vi "Voltage_Current.vi"() -> ()   [LabVIEW 2012]
uses:
  <instrlib>/Tektronix PWS4XXX Series/Tektronix PWS4XXX Series.lvlib
  <instrlib>/Tektronix DMM4020/Tektronix DMM4020.lvlib
panel:
  in  "stop":bool
  in  "Tab Control":T1(tab)
  in  "Step":dbl
  in  "Umin, V":dbl
  in  "Umax, V":dbl
  out "I, A":dbl format="%#.6f"
  out "U, V":dbl
  out "Current-Voltage Curve":cluster{dbl[], dbl[]}(graph)
  in  "Step, s":dbl
  in  "Seconds":dbl
  in  "Minutes":dbl
  in  "Hours":dbl
  in  "Value (V/A)":dbl format="%.2f"
  in  "Fixed function":u16(ring) items=["Voltage", "Current"]
  in  "Measurement Function":u16(ring) items=["DC Volts", "AC Volts", "DC Current", "AC Current", "2-Wire Resistance", "4-Wire Resistance", "Frequency", "AC and DC rms Current", "AC and DC rms Volts", "Continuity", "Diode"]
  out "Present value":dbl format="%#.6f"
  out "Unit":string
  out "Current-Voltage Curve 2":cluster{dbl[], dbl[]}(graph)
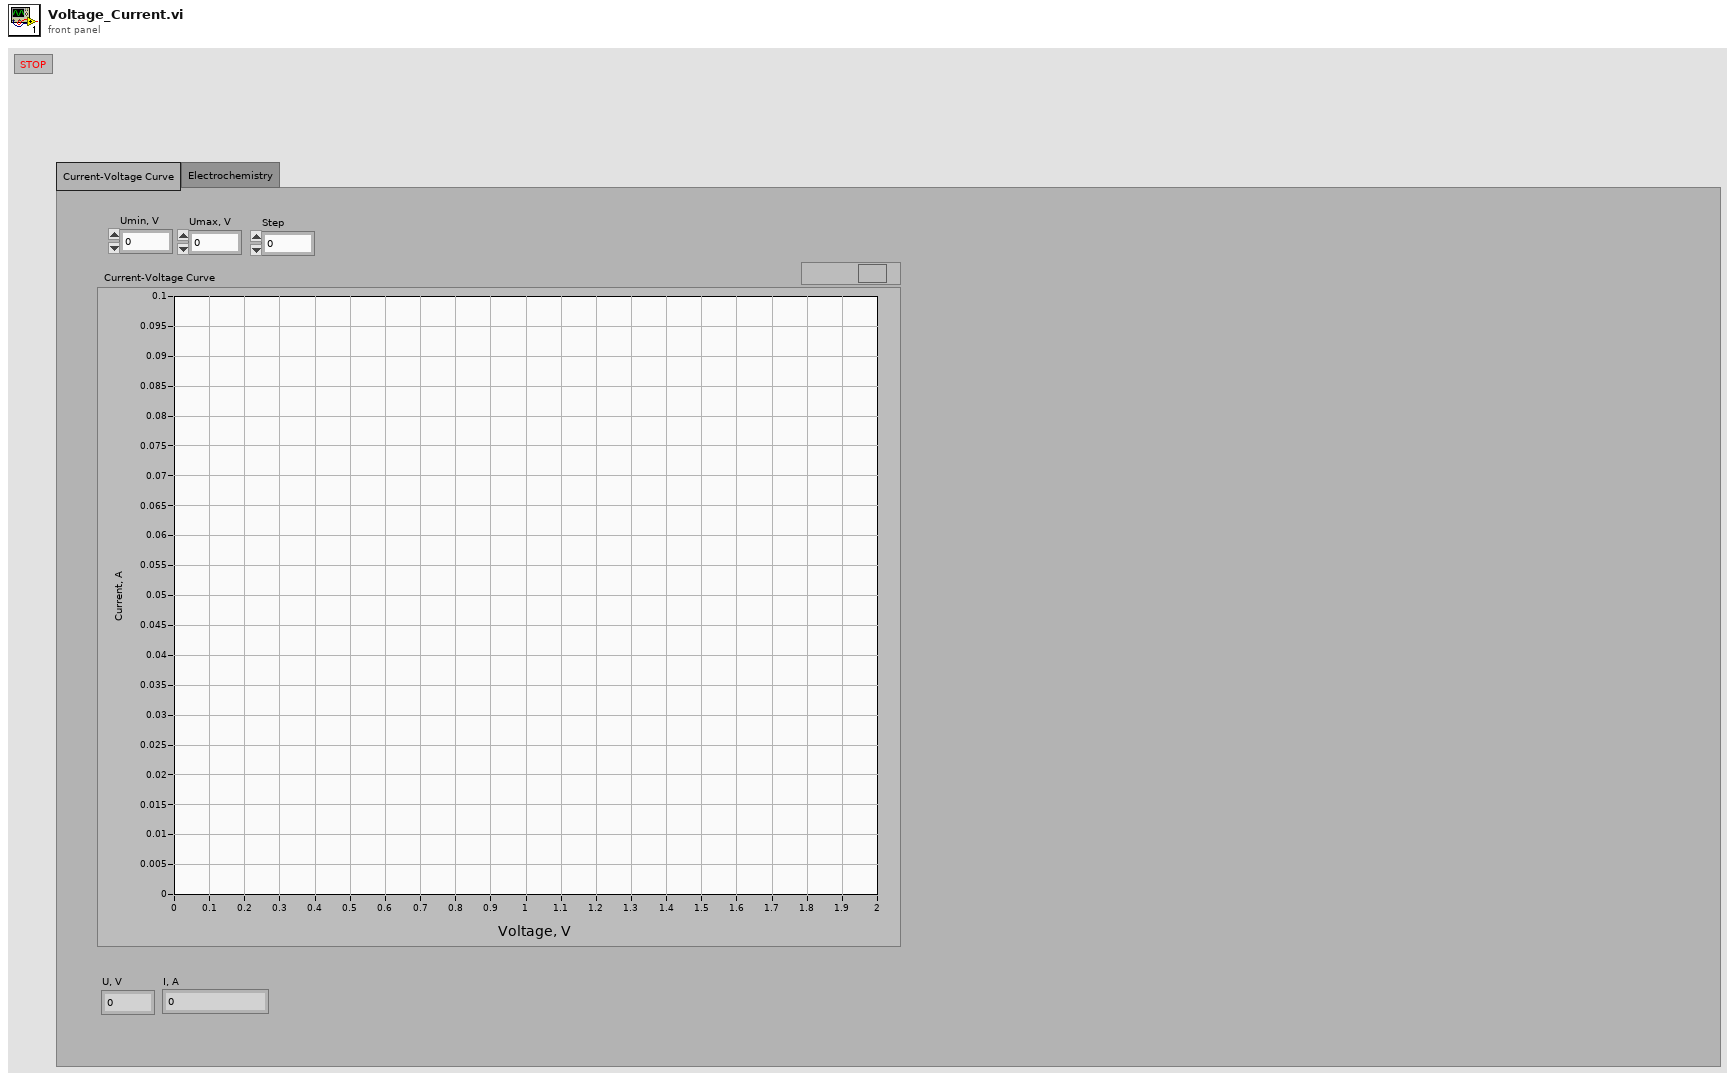
[diagram p1: front panel]
types:
  T1 = enum32{"Current-Voltage Curve", "Electrochemistry"}
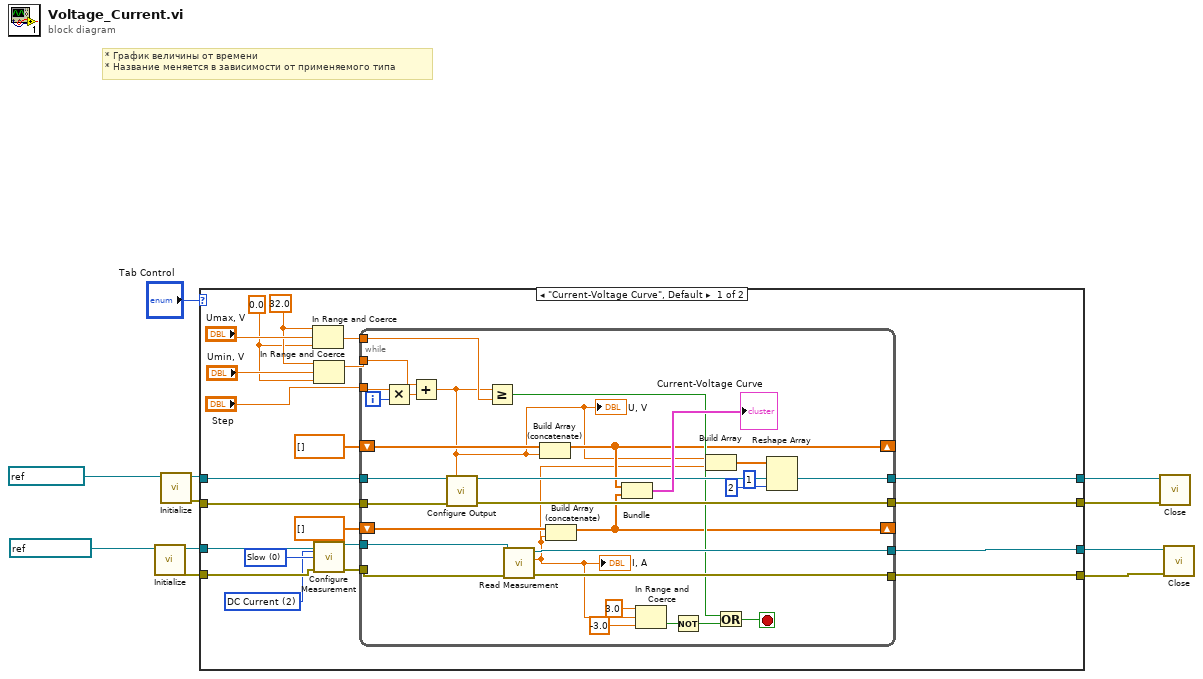
[diagram p0: block diagram]
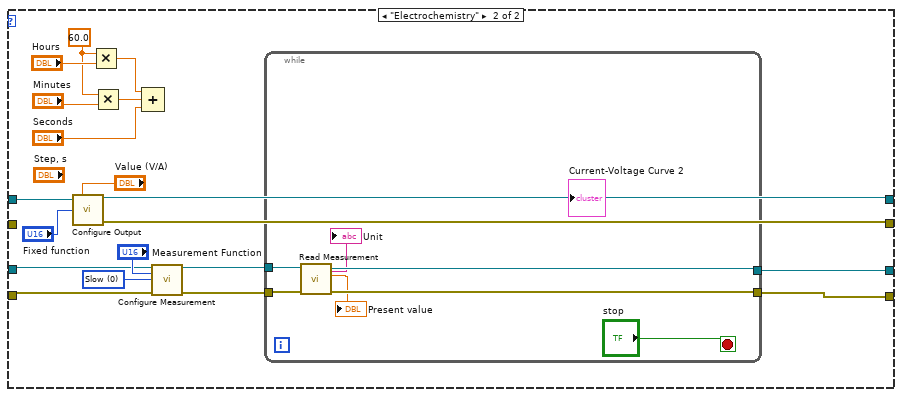
[diagram p2: hidden frame]
diagram:
  # "* График величины от времени\n* Название меняется в зависимости от применяемого типа"
  n1 = call <instrlib>:"Initialize.vi"("VISA resource name"=refnum<visa-resource-name> "DMM4020") -> ("error out"=w8:errorcluster, "VISA resource name out"=w9:refnum<visa-resource-name>)  [unwired: 9 in]
  n2 = call <instrlib>:"Initialize.vi"("VISA resource name"=refnum<visa-resource-name> "PWS4323") -> ("error out"=w2:errorcluster, "VISA resource name out"=w3:refnum<visa-resource-name>)  [unwired: 9 in]
  n3 = case shown="\"Current-Voltage Curve\", Default" "Tab Control" {
    tunnel: w3 -> [w25 w74]
    tunnel: w2 -> [w24 _]
    tunnel: w9 -> [w16 w67]
    tunnel: w8 -> [w15 w66]
    tunnel: [w23 w71] -> w7
    tunnel: [w22 w70] -> w6
    tunnel: [w21 w62] -> w5
    tunnel: [w20 w63] -> w4
    frame "Current-Voltage Curve", Default {
      w17 = u16 0 items=["Slow", "Medium", "Fast"] ("Measurement Rate (0: Slow)")
      w14 = u16 2 items=["DC Volts", "AC Volts", "DC Current", "AC Current", "2-Wire Resistance", "4-Wire Resistance", "Frequency", "AC and DC rms Current", "AC and DC rms Volts", "Continuity", "Diode"] ("Measurement Function (0: DC Volts)")
      w29 = 0.0 ("lower limit")
      w30 = 32.0 ("upper limit")
      n4 = In Range and Coerce(upper limit=w30, x="Umax, V", lower limit=w29) -> (coerced(x)=w26:dbl)  [unwired: 1 out]
      n5 = In Range and Coerce(upper limit=w30, x="Umin, V", lower limit=w29) -> (coerced(x)=w27:dbl)  [unwired: 1 out]
      n6 = call <instrlib>:"Configure Measurement.vi"("VISA resource name"=w16, "Measurement Function (0: DC Volts)"=w14, "Measurement Rate (0: Slow)"=w17, "error in (no error)"=w15) -> ("VISA resource name out"=w13:refnum<visa-resource-name>, "error out"=w12:errorcluster)  [unwired: 10 in]
      n7 = while {
        tunnel: "Step" -> [w60]
        tunnel: w27 -> [w58]
        tunnel: w26 -> [w57]
        tunnel: w25 -> [w56]
        tunnel: w24 -> [w55]
        shift-right: [w41] -> _
        shift-left: dbl[] [] -> [w47]
        shift-right: [w40] -> _
        shift-left: dbl[] [] -> [w46]
        tunnel: [w53] -> w23
        tunnel: [w52] -> w22
        tunnel: [w51] -> w21
        tunnel: [w50] -> w20
        tunnel: w13 -> [w34]
        tunnel: w12 -> [w33]
        i -> [w61]
        stop <- w49 stop-if-true
        n8 = Multiply(x=w60, y=w61) -> (x*y=w59:dbl)
        n9 = Add(x=w58, y=w59) -> (x+y=w39:dbl)
        "U, V" <- w39
        n10 = call <instrlib>:"Configure Output.vi"("VISA resource name"=w56, "Manual Range(0.00)"=w39, "error in (no error)"=w55) -> ("VISA resource name out"=w53:refnum<visa-resource-name>, "error out"=w52:errorcluster)  [unwired: 11 in]
        n11 = Greater Or Equal?(x=w39, y=w57) -> (x >= y?=w48:bool)
        n12 = call <instrlib>:"Read Measurement.vi"("error in (no error)"=w33, "VISA resource name"=w34) -> ("error out"=w50:errorcluster, "Primary Display Measurement"=w38:dbl, "VISA resource name out"=w51:refnum<visa-resource-name>)  [unwired: 4 in, 3 out]
        "I, A" <- w38
        n13 = Build Array (concatenate)(w47, w39) -> (w41:dbl[])
        n14 = Build Array (concatenate)(w46, w38) -> (w40:dbl[])
        n15 = Bundle(w41, w40) -> (→"Current-Voltage Curve":cluster{dbl[], dbl[]})  [unwired: 1 in]
        n16 = In Range and Coerce(upper limit=3.0 ("y"), x=w38, lower limit=-3.0) -> (In Range?=w43:bool)  [unwired: 1 out]
        n17 = Not(x=w43) -> (.not. x?=w42:bool)
        n18 = Build Array(w39, w38) -> (w37:dbl[])
        n19 = Or(x=w48, y=w42) -> (x .or. y?=w49:bool)
        n20 = Reshape Array(w37, 1 ("dimension size"), 2 ("dimension size")) -> ()  [unwired: 1 out]
      }
    }
    frame "Electrochemistry" {
      w69 = u16 0 items=["Slow", "Medium", "Fast"] ("Measurement Rate (0: Slow)")
      w78 = 60.0 ("y")
      n21 = call <instrlib>:"Configure Output.vi"("VISA resource name"=w74, "Manual Range(0.00)"="Value (V/A)", "Function(0:Voltage)"="Fixed function") -> ("VISA resource name out"=w71:refnum<visa-resource-name>, "error out"=w70:errorcluster)  [unwired: 11 in]
      n22 = Multiply(x=w78, y="Hours") -> (x*y=w77:dbl)
      n23 = Multiply(x=w78, y="Minutes") -> (x*y=w76:dbl)
      n24 = Compound Arithmetic op=ADD(w77, w76, "Seconds") -> ()  [unwired: 1 out]
      n25 = call <instrlib>:"Configure Measurement.vi"("VISA resource name"=w67, "Measurement Function (0: DC Volts)"="Measurement Function", "Measurement Rate (0: Slow)"=w69, "error in (no error)"=w66) -> ("VISA resource name out"=w65:refnum<visa-resource-name>, "error out"=w64:errorcluster)  [unwired: 10 in]
      n26 = while {
        tunnel: w65 -> [w86]
        tunnel: w64 -> [w85]
        tunnel: [w84] -> w63
        tunnel: [w83] -> w62
        stop <- "stop" stop-if-true
        n27 = call <instrlib>:"Read Measurement.vi"("error in (no error)"=w85, "VISA resource name"=w86) -> ("error out"=w84:errorcluster, "Primary Display Measurement"=→"Present value":dbl, "VISA resource name out"=w83:refnum<visa-resource-name>, "Primary Display Units"=→"Unit":string)  [unwired: 4 in, 2 out]
      }
    }
  }
  n28 = call <instrlib>:"Close.vi"("error in (no error)"=w6, "VISA resource name"=w7) -> ()  [unwired: 9 in, 1 out]
  n29 = call <instrlib>:"Close.vi"("error in (no error)"=w4, "VISA resource name"=w5) -> ()  [unwired: 9 in, 1 out]
